vi "Derivative Power BAP5.vi"(8 "Control Parameters":T1 {"Settle time" format="%.2f"; "Derivative time" format="%.2f"; "Integral time" format="%.2f"; "Settle bandwidth" format="%.2f"; "Control bandwidth" format="%.2f"; "Setpoint" format="%.2f"}, 9 "RESET":bool, 10 "elapsed time":dbl, 11 "Temp In (deg C)":dbl) -> (2 "Derivative Power":dbl)   [LabVIEW 2014]
doc: "Derivative Power BAP5\n\nCalculates the Derivative Power based off of Current Temperature (°C), Control Bandwidth (°C), Derivative Time (s), Elapsed Time (s), Derivative On, and RESET. RESET initializes the Derivative Power to 0.\n\nDerivative Power = -(Derivative Time / Control Bandwidth) * ((Current Temperature - Previous Temperature) / Elapsed Time), if Derivative On = True\n\n = 0, if Derivative On = False\n\nBeverly Abadines \nPHY 350"
uses:
  typedefs/control parameters.ctl
panel:
  # "Beverly Abadines\nPhys 350\nP5"
  # "Derivative Power"
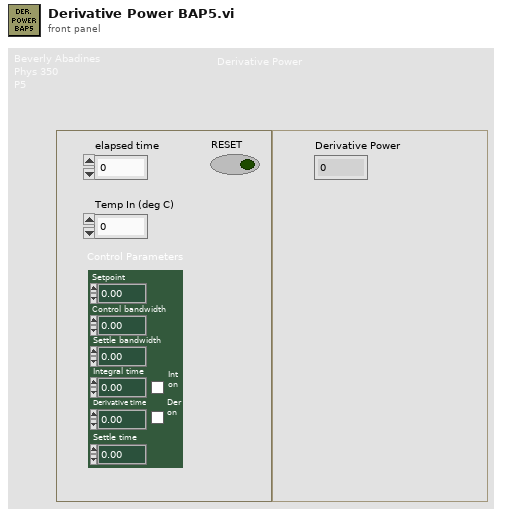
[diagram p1: front panel]
types:
  T1 = typedef "control parameters.ctl" = cluster{"Setpoint":dbl, "Control bandwidth":dbl, "Settle bandwidth":dbl, "Integral time":dbl, "Int\non":bool, "Derivative time":dbl, "Der\non":bool, "Settle time":dbl}
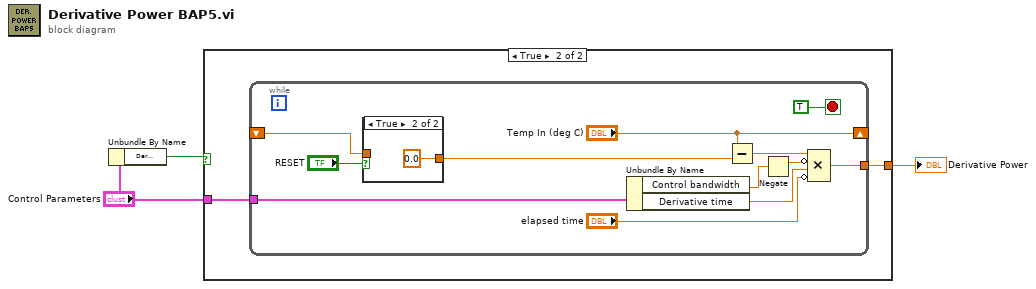
[diagram p0: block diagram]
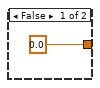
[diagram p2: hidden frame]
diagram:
  n1 = Unbundle By Name("Control Parameters") -> ("Der\non"=w1:bool)
  n2 = case shown="True" w1 {
    tunnel: [0.0 w6] -> w3
    tunnel: "Control Parameters" -> [_ w5]
    frame False {
    }
    frame True {
      n3 = while {
        shift-right: ["Temp In (deg C)"] -> _
        shift-left: _ -> [w11]
        tunnel: [w14] -> w6
        tunnel: w5 -> [w9]
        stop <- TRUE stop-if-true
        n4 = case shown="True" "RESET" {
          tunnel: [w19 0.0] -> w10
          tunnel: w11 -> [w19 _]
          frame False {
          }
          frame True {
          }
        }
        n5 = Unbundle By Name(w9) -> ("Control bandwidth"=w8:dbl, "Derivative time"=w15:dbl)
        n6 = Subtract(x="Temp In (deg C)", y=w10) -> (x-y=w17:dbl)
        n7 = Negate(x=w8) -> (-x=w7:dbl)
        n8 = Compound Arithmetic op=MULTIPLY(w17, invert w7, w15, invert "elapsed time") -> (w14:dbl)
      }
    }
  }
  "Derivative Power" <- w3
